vi "Main-COMinput.vi"() -> ()   [LabVIEW 2014]
uses:
  <vilib>/Instr/_visa.llb/VISA Set IO Buffer Mask.ctl
  <vilib>/Instr/_visa.llb/VISA Configure Serial Port (Instr).vi
panel:
  out "Receive\nPacket":bool
  in  "QueueName":string="ByteQueue"
  out "error out":errorcluster
  in  "stop":bool
  in  "size":u32=4096
  in  "Mask":T1=16 items=["I/O Receive Buffer"=16, "I/O Transmit Buffer"=32, "I/O Receive and Transmit Buffer"=48]
  in  "baud rate":u32=115200
  in  "data bits (8)":u16=8
  in  "parity (0:none)":enum16{"None", "Odd", "Even", "Mark", "Space"}(ring)
  in  "VISA resource name":refnum<visa-resource-name>
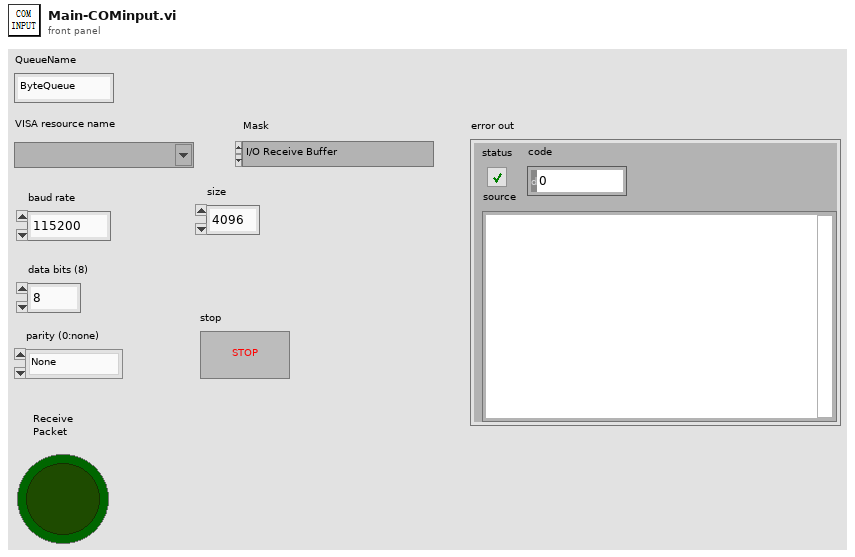
[diagram p1: front panel]
types:
  T1 = typedef "VISA Set IO Buffer Mask.ctl" = u16
  T2 = cluster{"Timestamp(4)":u32, "Sequence(4)":u32, "JY61ACC(2)":dbl[], "JY61GRY(3)":dbl[], "JY61AGL(3)":dbl[], "GY52ACC(2)":dbl[], "GY52GRY(3)":dbl[], "ADC1(3)":dbl[], "ADC2(3)":dbl[], "LFT/RAT":string}
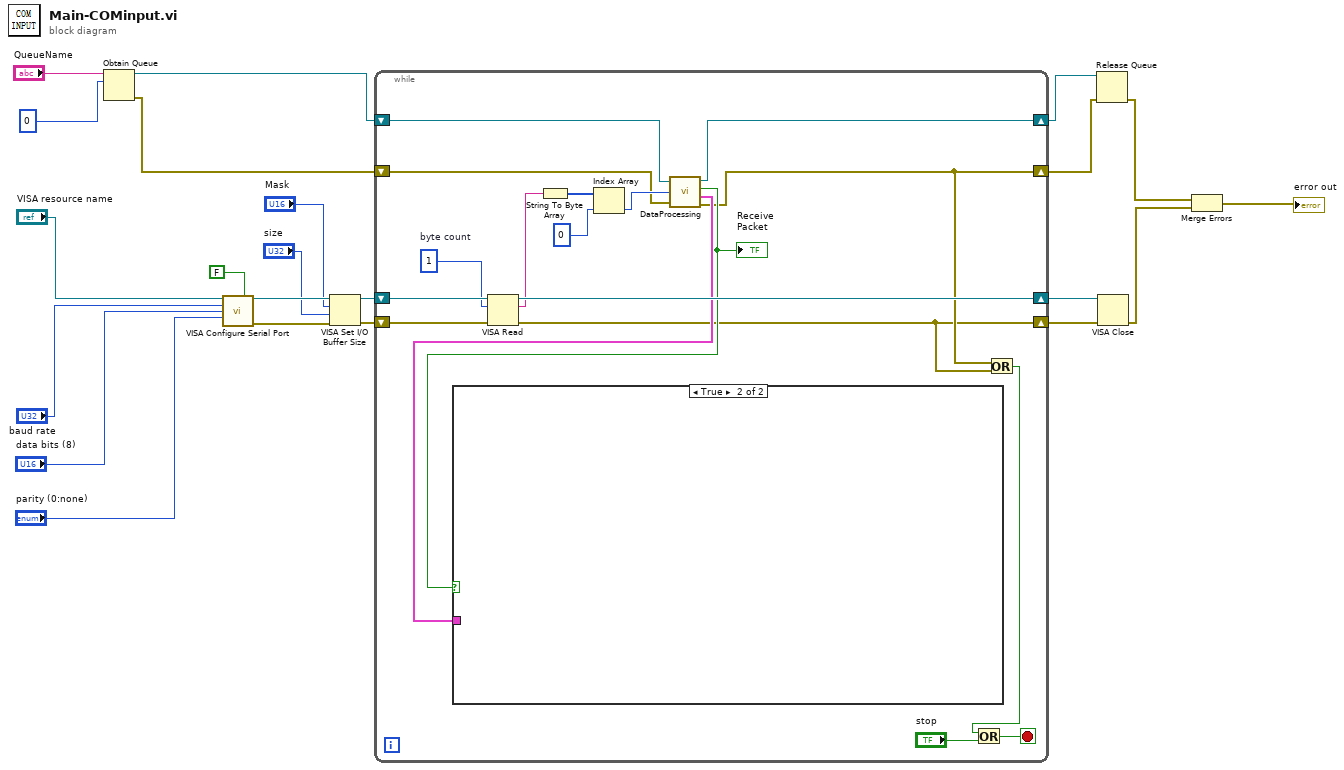
[diagram p0: block diagram]
diagram:
  n1 = Obtain Queue(name (unnamed)="QueueName", element data type=u8 0) -> (queue out=w8:refnum<queue>, error out=w5:errorcluster)  [unwired: 3 in, 1 out]
  n2 = call-poly "VISA Configure Serial Port"("VISA resource name"="VISA resource name", "Enable Termination\nChar (T)"=FALSE ("Enable Termination\nChar (T)"), "baud rate (9600)"="baud rate", "data bits (8)"="data bits (8)", "parity (0:none)"="parity (0:none)") -> ("VISA resource name out"=w17:refnum<visa-resource-name>, "error out"=w16:errorcluster)  [unwired: 9 in]
  n3 = VISA Set I/O Buffer Size(VISA resource name=w17, mask (16)="Mask", size (4096)="size", error in (no error)=w16) -> (VISA resource name out=w14:refnum<visa-resource-name>, error out=w13:errorcluster)
  n4 = while {
    shift-right: [w40] -> w15
    shift-left: w14 -> [w39]
    shift-right: [w32] -> w7
    shift-left: w8 -> [w34]
    shift-right: [w26] -> w6
    shift-left: w13 -> [w29]
    shift-right: [w27] -> w4
    shift-left: w5 -> [w28]
    stop <- w23 stop-if-true
    w33 = u32 1  # byte count
    n5 = VISA Read(VISA resource name=w39, byte count=w33, error in (no error)=w29) -> (VISA resource name out=w40:refnum<visa-resource-name>, read buffer=w36:string, error out=w26:errorcluster)  [unwired: 1 out]
    n6 = String To Byte Array(string=w36) -> (unsigned byte array=w37:u8[])
    n7 = Index Array(array=w37, index=0) -> (element=w35:u8)
    n8 = call "DataProcessing.vi"("queue in"=w34, "element"=w35, "error in"=w28) -> ("queue out"=w32:refnum<queue>, "Receive\nPacket"=w31:bool, "Message out"=w30:T2, "error out"=w27:errorcluster)
    "Receive\nPacket" <- w31
    n9 = case shown="True" w31 {
      tunnel: w30 -> [_ _]
      frame False {
      }
      frame True {
      }
    }
    n10 = Or(x=w27, y=w26) -> (x .or. y?=w24:bool)
    n11 = Or(x=w24, y="stop") -> (x .or. y?=w23:bool)
  }
  n12 = Release Queue(queue=w7, error in (no error)=w4) -> (error out=w3:errorcluster)  [unwired: 1 in, 2 out]
  n13 = VISA Close(VISA resource name=w15, error in (no error)=w6) -> (error out=w2:errorcluster)
  n14 = Merge Errors(w3, w2) -> (→"error out":errorcluster)
